vi "WriteRead Data.vi"(6 "NoStop (F)":bool, 7 "I2C Peripheral":refnum<class "I2C Connection.lvclass">, 8 "error in (no error)":errorcluster, 9 "Len":u8, 10 "Write Data":string) -> (0 "error out":errorcluster, 1 "Read Data":string)   [LabVIEW 2020, in "CTI.lvlib" / "I2C Connection.lvclass"]
uses:
  I2C Connection.lvclass
  I2C Connection.lvclass/I2C Connection.ctl
  Session/Session.lvclass
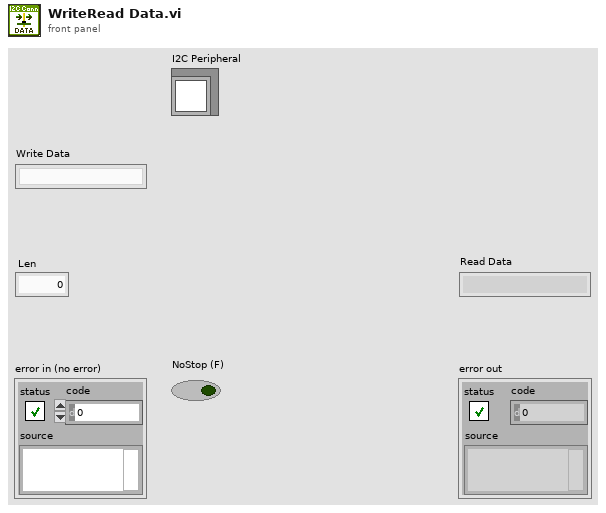
[diagram p1: front panel]
types:
  T1 = typedef "CTI.lvlib/I2C Address.ctl" = u8
  T2 = typedef "CTI.lvlib/I2C Number.ctl" = i8
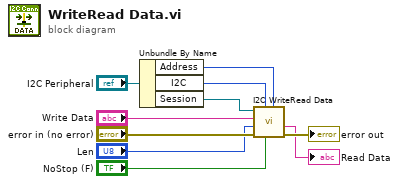
[diagram p0: block diagram]
diagram:
  n1 = Unbundle By Name("I2C Peripheral") -> ("Address"=w5:T1, "I2C"=w6:T2, "Session"=w1:refnum<class "Session.lvclass">)
  n2 = call "I2C WriteRead Data.vi"("Address"=w5, "NoStop (F)"="NoStop (F)", "I2C #"=w6, "error in (no error)"="error in (no error)", "Len"="Len", "Write Data"="Write Data", "Session in"=w1) -> ("error out"=→"error out":errorcluster, "Read Data"=→"Read Data":string)  [unwired: 2 in, 1 out]
